vi "tester.vi"() -> ()   [LabVIEW 2019]
uses:
  state.ctl
panel:
  in  "setpoints":T1={"target clarified turbidity (NTU)"=0.3, "flocculator volume (L)"=0.0, "clarifier volume (L)"=0.0, "updates per HRT"=1} {"target clarified turbidity (NTU)" min=0.1 max=5.0 step=0.01; "updates per HRT" min=1 step=1}
  out "setpoints out":T2
  in  "change setpoints":bool
  in  "stop":bool
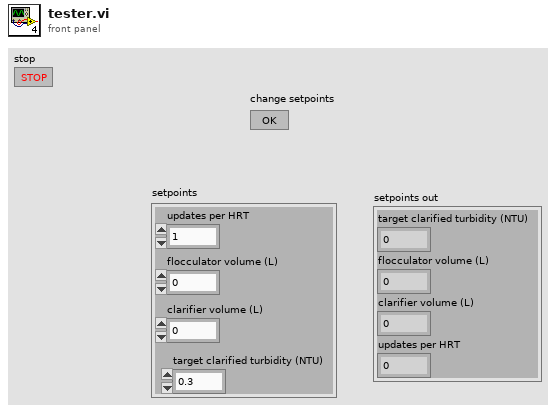
[diagram p1: front panel]
types:
  T1 = cluster{"target clarified turbidity (NTU)":dbl, "flocculator volume (L)":dbl, "clarifier volume (L)":dbl, "updates per HRT":u32}
  T2 = cluster{"target clarified turbidity (NTU)":dbl, "flocculator volume (L)":dbl, "clarifier volume (L)":dbl, "updates per HRT":dbl}
  T3 = typedef "state.ctl" = enum16{"Initialize", "Change setpoints", "Process data", "Close"}
  T4 = typedef "setpoints.ctl" = cluster{"target clarified turbidity (NTU)":dbl, "flocculator volume (L)":dbl, "clarifier volume (L)":dbl, "dose updates per HRT":u32}
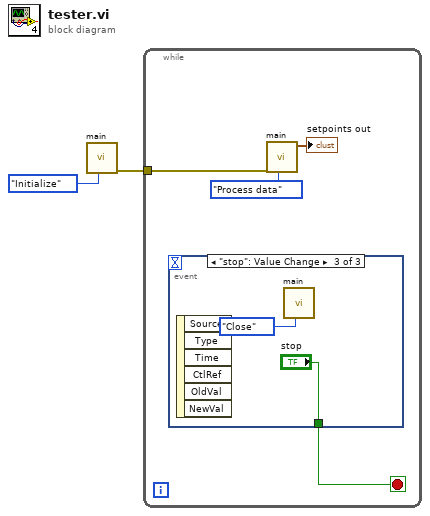
[diagram p0: block diagram]
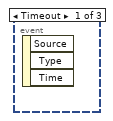
[diagram p2: hidden frame]
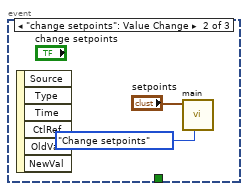
[diagram p3: hidden frame]
diagram:
  n1 = call "main.vi"("Enum"=state."Initialize") -> ("error out"=w2:errorcluster)  [unwired: 9 in, 1 out]
  n2 = while {
    tunnel: w2 -> [w6]
    stop <- w3 stop-if-true
    n3 = event shown="[2] \"stop\": Value Change" {
      selector: _ -> [_ _ _]
      dyn-events: _ -> [_ _ _]
      timeout: _ -> [_ _ _]
      tunnel: [_ _ "stop"] -> w3
      event Timeout {
        n4 = event-data() -> ()  [unwired: 1 in, 3 out]
      }
      event "change setpoints": Value Change {
        n5 = event-data() -> ()  [unwired: 1 in, 6 out]
        n6 = call "main.vi"("Enum"=state."Change setpoints", "setpoints"="setpoints") -> ()  [unwired: 8 in, 2 out]
      }
      event "stop": Value Change {
        n7 = event-data() -> ()  [unwired: 1 in, 6 out]
        n8 = call "main.vi"("Enum"=state."Close") -> ()  [unwired: 9 in, 2 out]
      }
    }
    n9 = call "main.vi"("Enum"=state."Process data", "error in (no error)"=w6) -> ("setpoints out"=→"setpoints out":T4)  [unwired: 8 in, 1 out]
  }
